vi "Read Set Trigger.vi"(8 "error in (no error)":errorcluster, 11 "Simulated_CCD_Camera in":refnum<class "Simulated_CCD_Camera.lvclass">) -> (0 "error out":errorcluster, 2 "Set Trigger":bool, 3 "Simulated_CCD_Camera out":refnum<class "Simulated_CCD_Camera.lvclass">)   [LabVIEW 2018, in "Simulated_CCD_Camera.lvclass"]
uses:
  Simulated_CCD_Camera.lvclass
  Simulated_CCD_Camera.lvclass/Simulated_CCD_Camera.ctl
  Interface/Interface.lvclass
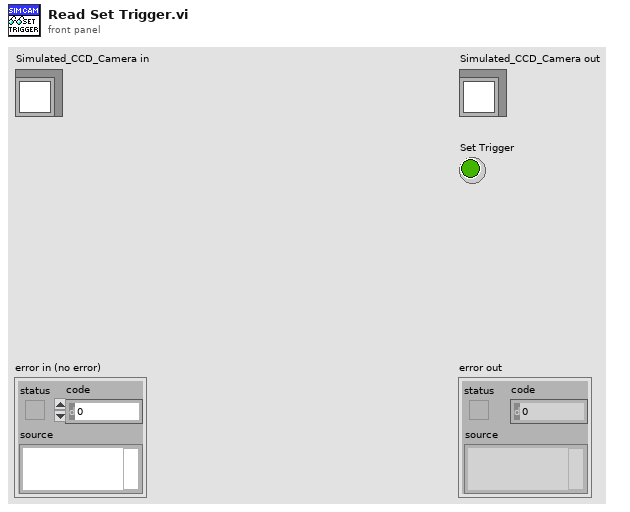
[diagram p1: front panel]
types:
  T1 = cluster{"Exposure Time":sgl, "Pre-amp gain":u8, "Readout Rate":u8, "EM Mode":u8, "EM Gain":u16, "Binning":u16, "Initial Line":u16, "Initial Cloumn":u16, "Final Line":u16, "Final Column":u16, "Kinetic Series Length":u32, "Shutter Mode":u8, "Cooler ON/OFF":u16, "Temperature":i8, "Cubes":u32, "Trigger":u16, "Set Trigger":bool}
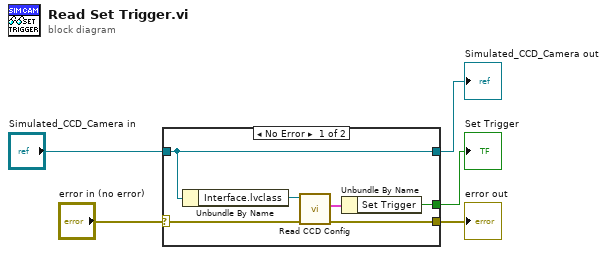
[diagram p0: block diagram]
diagram:
  n1 = case shown="No Error" "error in (no error)" {
    selector: "error in (no error)" -> [w9 w12]
    tunnel: [w10 w12] -> w4
    tunnel: [w11 w13] -> w2
    tunnel: "Simulated_CCD_Camera in" -> [w11 w13]
    tunnel: [w6 _] -> w1
    frame No Error {
      n2 = Unbundle By Name(w11) -> ("Interface.lvclass"=w8:refnum<class "Interface.lvclass">)
      n3 = call "Read CCD Config.vi"("error in (no error)"=w9, "Interface in"=w8) -> ("error out"=w10:errorcluster, "CCD Config"=w7:T1)  [unwired: 7 in, 1 out]
      n4 = Unbundle By Name(w7) -> ("Set Trigger"=w6:bool)
    }
    frame Error {
    }
  }
  "error out" <- w4
  "Simulated_CCD_Camera out" <- w2
  "Set Trigger" <- w1
